vi "DblMonoPMDCurrentScan.vi"() -> ()   [LabVIEW 2009]
uses:
  <vilib>/DAQmx/create/channels.llb/DAQmx Create Channel (AI-Voltage-Basic).vi
  <vilib>/DAQmx/create/channels.llb/DAQmx Create Channel (AO-Voltage-Basic).vi
  <vilib>/DAQmx/write.llb/DAQmx Write (Analog DBL 1Chan 1Samp).vi
  <vilib>/DAQmx/read.llb/DAQmx Read (Analog 1D DBL 1Chan NSamp).vi
  <vilib>/DAQmx/configure/timing.llb/DAQmx Timing (Sample Clock).vi
  <vilib>/Utility/file.llb/Write To Spreadsheet File (DBL).vi
  <vilib>/Analysis/NI_AALBase.lvlib
panel:
  in  "PM Channel":refnum<visa-resource-name>="USB0::0x1313::0x8072::P2000362::INSTR"
  in  "Voltage B":dbl min=-10.0 max=10.0 step=0.1 format="%0.2f"
  in  "Voltage A":dbl min=-10.0 max=10.0 step=0.1 format="%0.2f"
  in  "Output B":tag="Dev1/ao3"
  in  "Output A":tag="Dev1/ao2"
  in  "Input Channel":tag="Dev1/ai6"
  in  "Current":bool
  in  "Power":bool=TRUE
  out "ScanGraph":cluster{dbl[], dbl[]}(graph)
  in  "Sensitivity":dbl=1e-09 caption="(A/V)" format="%#_6p"
  out "Readout":dbl=-5.1512643e-06 format="%^#_9e"
  in  "Scan Save Path":path
  in  "On":bool=TRUE
  out "Waveform Chart":dbl(graph)=-5.1512643e-06
  in  "Save":bool=TRUE
  in  "Exit":bool
  in  "STOP":bool
  in  "Step Time (sec)":dbl=1.0 min=0.001 max=300.0 step=0.001 format="%.3f"
  in  "Step Size (nm)":dbl=1.0 min=0.1 max=100.0 step=0.1 format="%.1f"
  in  "End":dbl=800.0 min=0.0 max=2000.0 step=0.1 format="%.1f"
  in  "Start":dbl=400.0 min=0.0 max=2000.0 step=0.1 format="%.1f"
  in  "Scan":bool
  in  "Up":bool=TRUE caption="Down"
  in  "Increment (nm)":dbl=10.0 min=0.1 max=2000.0 step=0.1 format="%.1f"
  in  "PMD Settings":T1={"Beam Diameter (mm)"=4.0, "BWIn"=0, "Averaging Rate"=300, "Auto Range"=TRUE} {"Averaging Rate" min=33 max=5000 step=1; "BWIn" items=["HIGH", "LOW"]; "Beam Diameter (mm)" min=1.0 max=9.0 step=0.5}
  in  "Step":bool
  out "Busy":bool
  in  "Send Command":bool
  in  "Command":u16(ring)=1 items=["nm", "goto", "nm/min", "VIS grating", "IR grating"]
  in  "Wavelength (nm)":dbl=500.0 min=0.0 max=2000.0 step=0.1 format="%.1f"
  in  "Scan Speed (nm/min)":dbl=100.0 min=1.0 max=500.0 step=0.1 format="%.1f"
  out "Done?":string="   ..."
  in  "Send Question":bool
  in  "Ask?":u16(ring) items=["?nm", "?nm/min", "?grating", "?turret", "?gratings"]
  in  "Zero?":bool
  out "PM Error log":string
  out "AUTO?":bool
  out "Zero Value":dbl format="%#.3p"
  out "Rng":string
  in  "Range":i16=1 min=1 max=6 step=1
  in  "Mono Port":refnum<visa-resource-name>="COM11"
  out "IDN String":string="Thorlabs,PM100USB,P2000362,1.3.0\n"
  out "Sensor SN":string="10061433"
  out "Sensor Name":string="S120C"
  out "Reply":string=" 0.000 nm  ok\r\n" caption="Mono Response"
  # "Range Settings"
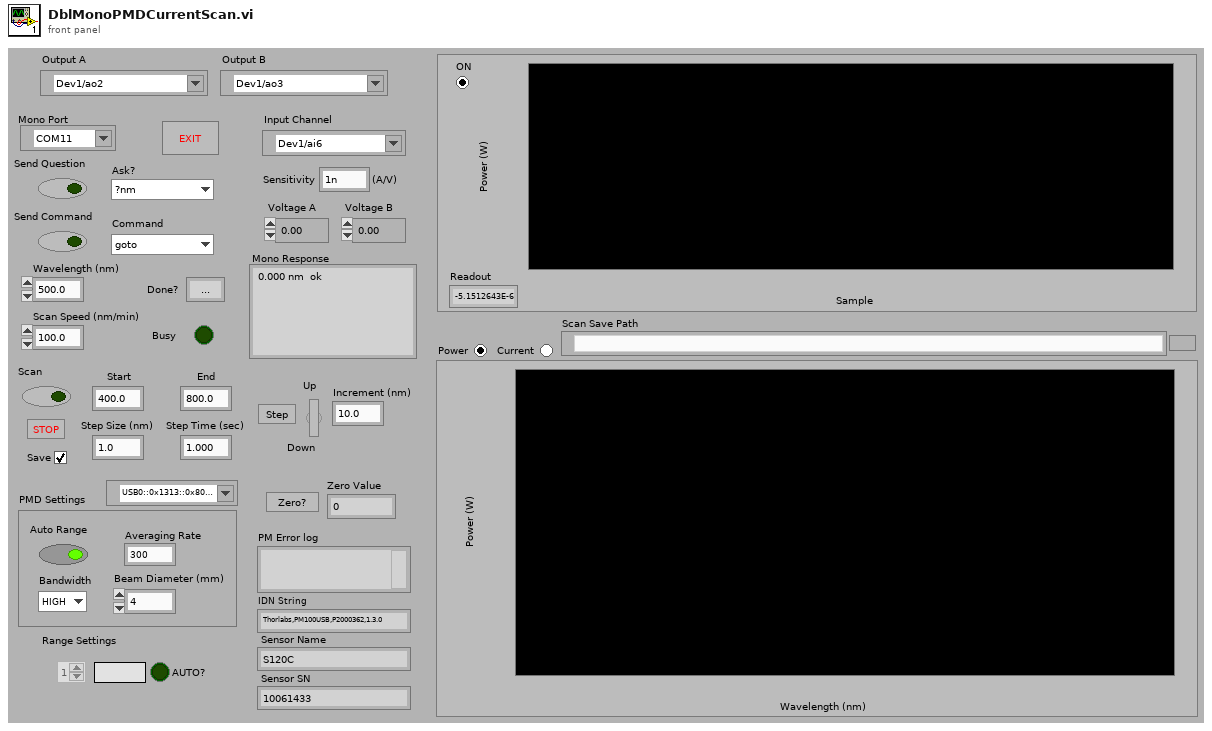
[diagram p1: front panel]
types:
  T1 = cluster{"Beam Diameter (mm)":dbl, "BWIn":u16, "Averaging Rate":i32, "Auto Range":bool}
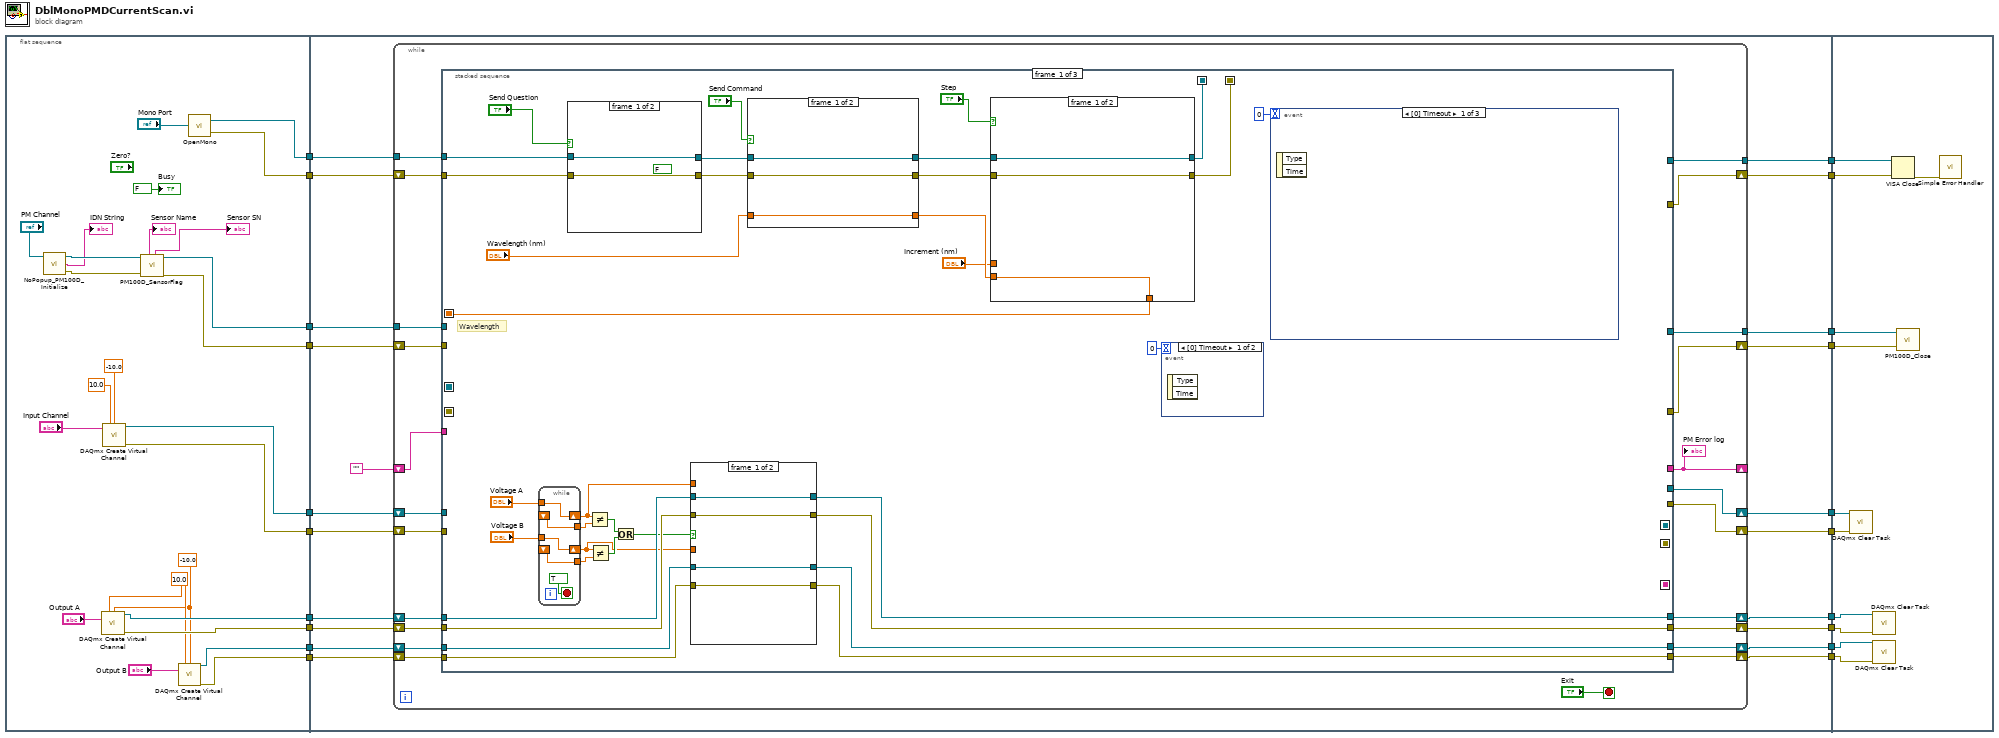
[diagram p0: block diagram]
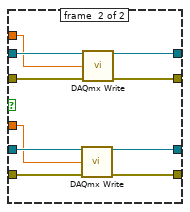
[diagram p2: hidden frame]
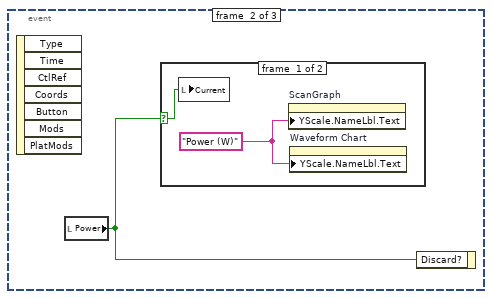
[diagram p3: hidden frame]
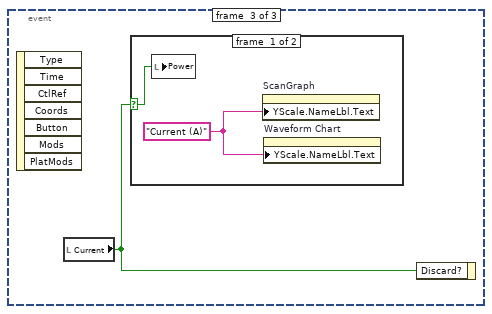
[diagram p5: hidden frame]
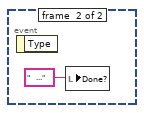
[diagram p7: hidden frame]
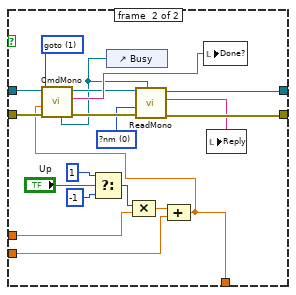
[diagram p8: hidden frame]
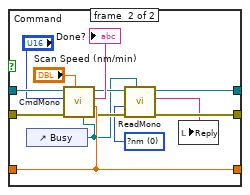
[diagram p9: hidden frame]
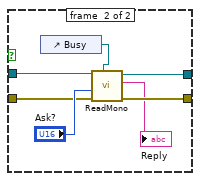
[diagram p10: hidden frame]
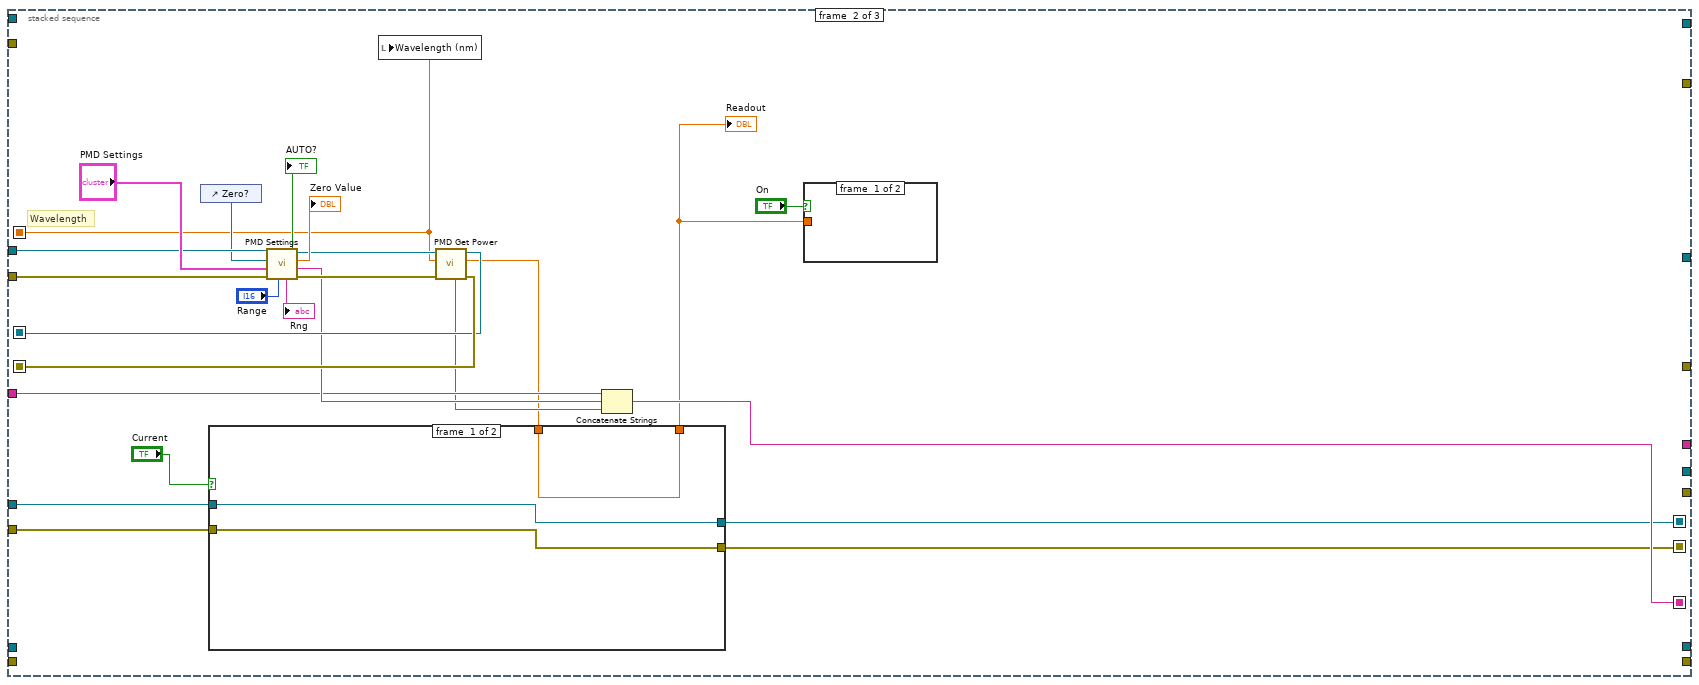
[diagram p11: hidden frame]
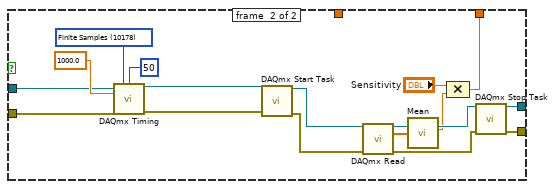
[diagram p12: hidden frame]
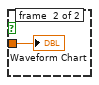
[diagram p13: hidden frame]
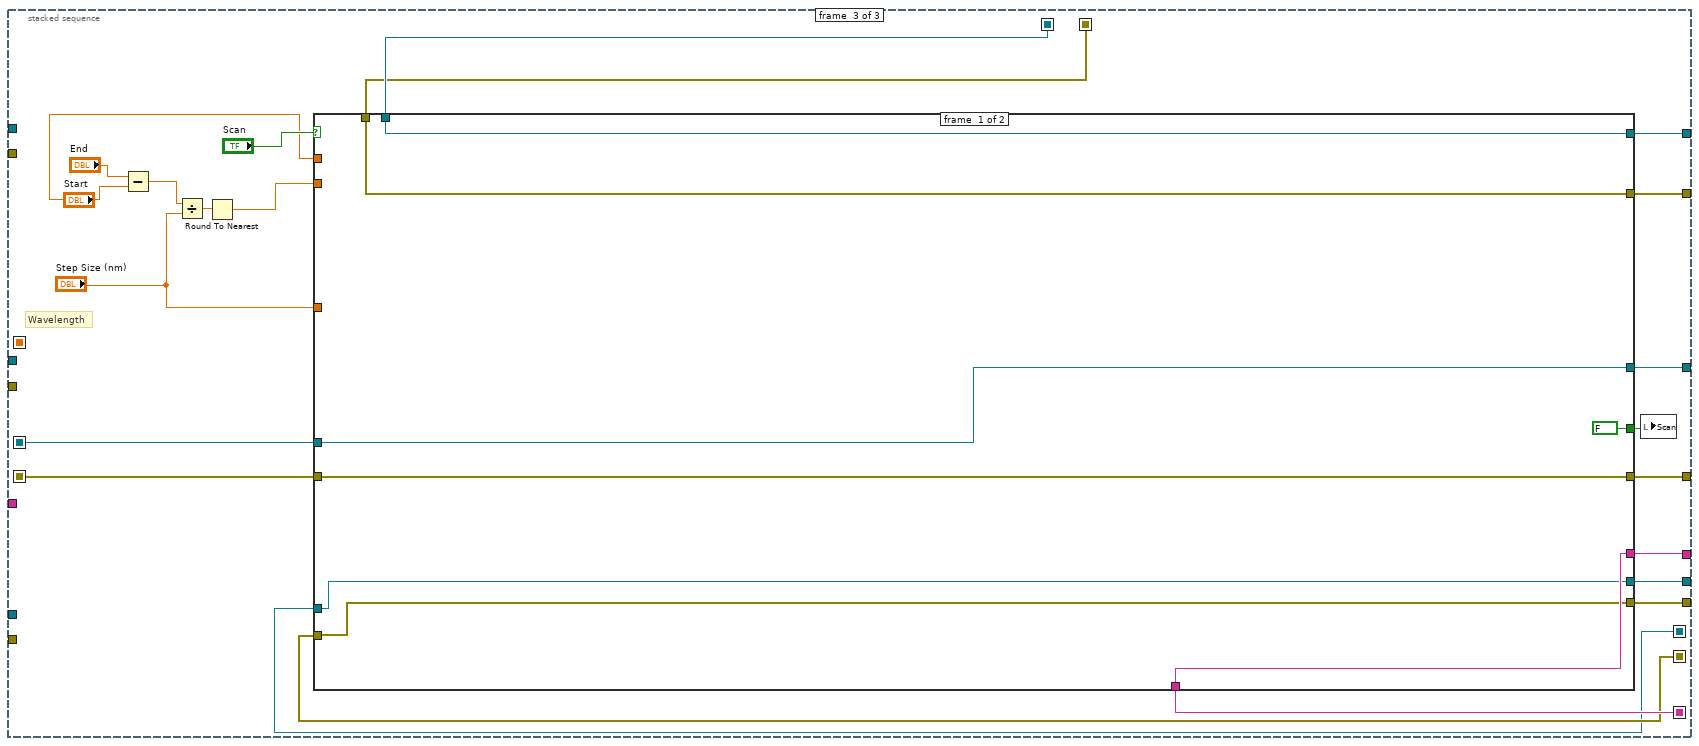
[diagram p14: hidden frame]
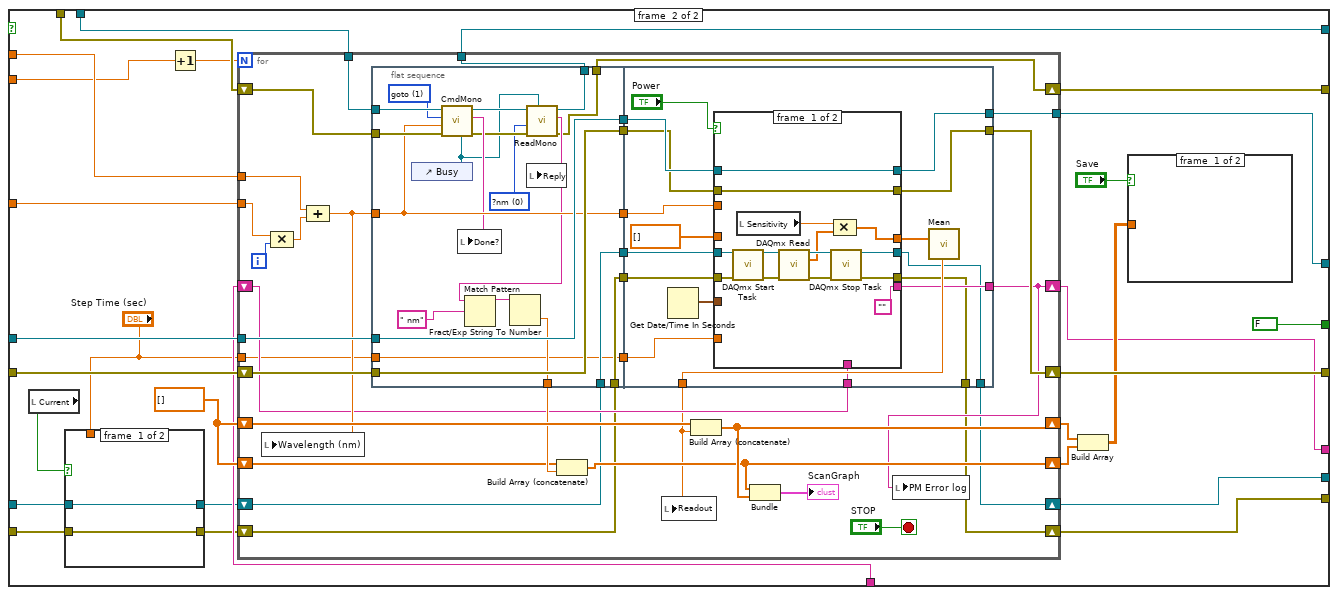
[diagram p15: hidden frame]
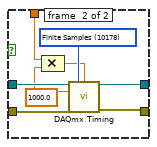
[diagram p16: hidden frame]
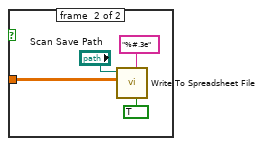
[diagram p17: hidden frame]
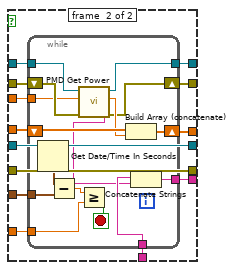
[diagram p18: hidden frame]
diagram:
  n1 = flat-sequence {
    tunnel: [w43] -> w20
    tunnel: [w42] -> w19
    tunnel: [w41] -> w18
    tunnel: [w40] -> w17
    tunnel: [w27] -> w12
    tunnel: [w28] -> w9
    tunnel: [w33] -> w8
    tunnel: [w34] -> w7
    tunnel: [w32] -> w6
    tunnel: [w31] -> w5
    tunnel: w20 -> [w65]
    tunnel: w19 -> [w66]
    tunnel: w18 -> [w64]
    tunnel: w17 -> [w63]
    tunnel: [w62] -> w16
    tunnel: [w61] -> w15
    tunnel: [w60] -> w14
    tunnel: [w59] -> w13
    tunnel: w12 -> [w56]
    tunnel: [w47] -> w11
    tunnel: [w46] -> w10
    tunnel: w9 -> [w57]
    tunnel: w8 -> [w55]
    tunnel: w7 -> [w54]
    tunnel: w6 -> [w53]
    tunnel: w5 -> [w52]
    tunnel: [w48] -> w4
    tunnel: [w49] -> w3
    tunnel: [w50] -> w2
    tunnel: [w51] -> w1
    tunnel: w16 -> [w438]
    tunnel: w15 -> [w437]
    tunnel: w14 -> [w436]
    tunnel: w13 -> [w435]
    tunnel: w11 -> [w433]
    tunnel: w10 -> [w434]
    tunnel: w4 -> [w432]
    tunnel: w3 -> [w431]
    tunnel: w2 -> [w430]
    tunnel: w1 -> [w429]
    frame #0 {
      w29 = -10.0 ("minimum value")
      w30 = 10.0 ("maximum value")
      n2 = call "NoPopup_PM100D_Initialize.vi"("PM Channel"="PM Channel") -> ("error out"=w23:errorcluster, "Instrument"=→"IDN String":string, "VISA out"=w24:refnum<visa-resource-name>)  [unwired: 1 in, 1 out]
      n3 = call-poly <vilib>:"DAQmx Create Virtual Channel.vi"("maximum value"=w30, "minimum value"=w29, "physical channels"="Output A") -> ("task out"=w34:refnum<k21>, "error out"=w33:errorcluster)  [unwired: 11 in]
      n4 = call-poly <vilib>:"DAQmx Create Virtual Channel.vi"("maximum value"=10.0, "minimum value"=-10.0, "physical channels"="Input Channel") -> ("task out"=w28:refnum<k21>, "error out"=w27:errorcluster)  [unwired: 11 in]
      n5 = call "PM100D_SensorFlag.vi"("error in (no error)"=w23, "VISA in"=w24) -> ("error out"=w43:errorcluster, "VISA out"=w42:refnum<visa-resource-name>, "sn"=→"Sensor SN":string, "name"=→"Sensor Name":string)  [unwired: 2 in, 4 out]
      n6 = call-poly <vilib>:"DAQmx Create Virtual Channel.vi"("maximum value"=w30, "minimum value"=w29, "physical channels"="Output B") -> ("task out"=w31:refnum<k21>, "error out"=w32:errorcluster)  [unwired: 11 in]
      n7 = call "OpenMono.vi"("Mono Port"="Mono Port") -> ("VISA resource name out"=w41:refnum<visa-resource-name>, "error out"=w40:errorcluster)
      "Busy" <- FALSE ("Busy")
    }
    frame #1 {
      n8 = while {
        tunnel: w66 -> [w87]
        tunnel: w64 -> [w89]
        tunnel: [w84] -> w61
        tunnel: [w82] -> w59
        shift-right: [w81] -> w60
        shift-left: w65 -> [w86]
        shift-right: [w83] -> w62
        shift-left: w63 -> [w88]
        shift-right: [w79] -> _
        shift-left: "" -> [w80]
        shift-right: [w68] -> w46
        shift-left: w56 -> [w77]
        shift-right: [w67] -> w47
        shift-left: w57 -> [w78]
        shift-right: [w69] -> w51
        shift-left: w54 -> [w76]
        shift-right: [w70] -> w50
        shift-left: w55 -> [w75]
        shift-right: [w71] -> w49
        shift-left: w52 -> [w73]
        shift-right: [w72] -> w48
        shift-left: w53 -> [w74]
        stop <- "Exit" stop-if-true
        n9 = stacked-sequence {
          seq-local: [w108 _ _] -> [_ w204 _]
          seq-local: [w113 _ _] -> [_ _ w257]
          seq-local: [w112 _ _] -> [_ _ w256]
          seq-local: [_ w211 _] -> [_ _ w255]
          seq-local: [_ w212 _] -> [_ _ w254]
          seq-local: [_ w205 _] -> [_ _ w248]
          seq-local: [_ w199 _] -> [_ _ w244]
          seq-local: [_ w200 _] -> [_ _ w243]
          tunnel: w89 -> [w119 _ _]
          tunnel: w88 -> [w118 _ _]
          tunnel: w87 -> [_ w214 _]
          tunnel: w86 -> [_ w213 _]
          tunnel: [_ _ w253] -> w84
          tunnel: [_ _ w252] -> w83
          tunnel: [_ _ w251] -> w82
          tunnel: [_ _ w250] -> w81
          tunnel: w80 -> [_ w207 _]
          tunnel: [_ _ w247] -> w79
          tunnel: w78 -> [_ w198 _]
          tunnel: w77 -> [_ w197 _]
          tunnel: [_ _ w246] -> w67
          tunnel: [_ _ w245] -> w68
          tunnel: w76 -> [w103 _ _]
          tunnel: w75 -> [w104 _ _]
          tunnel: w74 -> [w106 _ _]
          tunnel: w73 -> [w105 _ _]
          tunnel: [w102 _ _] -> w72
          tunnel: [w101 _ _] -> w71
          tunnel: [w100 _ _] -> w70
          tunnel: [w99 _ _] -> w69
          frame #0 {
            # "Wavelength"
            n10 = while {
              shift-right: [w141] -> w90
              shift-left: _ -> [w140]
              tunnel: "Voltage B" -> [w141]
              tunnel: [w140] -> w95
              tunnel: "Voltage A" -> [w139]
              shift-right: [w139] -> w91
              shift-left: _ -> [w138]
              tunnel: [w138] -> w96
              stop <- TRUE stop-if-true
            }
            n11 = case shown="True" "Send Question" {
              tunnel: w119 -> [w189 w195]
              tunnel: w118 -> [w188 w194]
              tunnel: [w189 w193] -> w121
              tunnel: [w188 w192] -> w120
              frame #0 {
                (unwired) FALSE ("Read Error")
              }
              frame #1 {
                n12 = control-ref of="Busy"() -> (w190:refnum<vi>)
                n13 = call "ReadMono.vi"("Busy"=w190, "error in (no error)"=w194, "Cmd"="Ask?", "Mono Port"=w195) -> ("error out"=w192:errorcluster, "Response"=→"Reply":string, "Mono Port Out"=w193:refnum<visa-resource-name>)  [unwired: 2 in, 1 out]
              }
            }
            n14 = Not Equal?(x=w91, y=w96) -> (x != y?=w94:bool)
            n15 = Not Equal?(x=w90, y=w95) -> (x != y?=w93:bool)
            n16 = Or(x=w94, y=w93) -> (x .or. y?=w92:bool)
            n17 = case shown="True" w92 {
              tunnel: w106 -> [w124 w137]
              tunnel: w105 -> [w125 w136]
              tunnel: w104 -> [w126 w135]
              tunnel: w103 -> [w127 w134]
              tunnel: [w124 w133] -> w102
              tunnel: [w125 w132] -> w101
              tunnel: [w126 w131] -> w100
              tunnel: [w127 w130] -> w99
              tunnel: w91 -> [_ w128]
              tunnel: w90 -> [_ w129]
              frame #0 {
              }
              frame #1 {
                n18 = call-poly <vilib>:"DAQmx Write.vi"("task/channels in"=w136, "data"=w129, "error in"=w137) -> ("task out"=w132:refnum<k21>, "error out"=w133:errorcluster)  [unwired: 10 in, 1 out]
                n19 = call-poly <vilib>:"DAQmx Write.vi"("task/channels in"=w134, "data"=w128, "error in"=w135) -> ("task out"=w130:refnum<k21>, "error out"=w131:errorcluster)  [unwired: 10 in, 1 out]
              }
            }
            n20 = case shown="True" "Send Command" {
              tunnel: w121 -> [w174 w187]
              tunnel: w120 -> [w173 w186]
              tunnel: [w174 w179] -> w116
              tunnel: [w173 w178] -> w115
              tunnel: "Wavelength (nm)" -> [w172 w182]
              tunnel: [w172 w182] -> w114
              frame #0 {
              }
              frame #1 {
                w177 = u16 0 items=["?nm", "?nm/min", "?grating", "?turret", "?gratings"] ("Cmd")
                n21 = control-ref of="Busy"() -> (w175:refnum<vi>)
                n22 = call "CmdMono.vi"("Busy"=w175, "Scan Speed (nm/min)"="Scan Speed (nm/min)", "error in (no error)"=w186, "Wavelength (nm)"=w182, "Cmd"="Command", "Mono Port"=w187) -> ("error out"=w180:errorcluster, "Response"=→"Done?":string, "Mono Port Out"=w181:refnum<visa-resource-name>)  [unwired: 2 in, 1 out]
                n23 = call "ReadMono.vi"("Busy"=w175, "error in (no error)"=w180, "Cmd"=w177, "Mono Port"=w181) -> ("error out"=w178:errorcluster, "Response"=w176:string, "Mono Port Out"=w179:refnum<visa-resource-name>)  [unwired: 2 in, 1 out]
                n24 = local write "Reply"(w176) -> ()
              }
            }
            n25 = case shown="False" "Step" {
              tunnel: w116 -> [w152 w171]
              tunnel: w115 -> [w151 w170]
              tunnel: w114 -> [w150 w164]
              tunnel: [w152 w157] -> w113
              tunnel: [w151 w158] -> w112
              tunnel: "Increment (nm)" -> [_ w163]
              tunnel: [w150 w153] -> w108
              frame #0 {
              }
              frame #1 {
                w155 = u16 0 items=["?nm", "?nm/min", "?grating", "?turret", "?gratings"] ("Cmd")
                w162 = u16 1 items=["nm", "goto", "nm/min", "VIS grating", "IR grating"] ("Cmd")
                n26 = Select(t=1, s="Up", f=-1) -> (s? t:f=w169:i32)
                n27 = control-ref of="Busy"() -> (w154:refnum<vi>)
                n28 = Compound Arithmetic op=MULTIPLY(w169, w163) -> (w165:dbl)
                n29 = Compound Arithmetic op=ADD(w165, w164) -> (w153:dbl)
                n30 = call "CmdMono.vi"("Busy"=w154, "error in (no error)"=w170, "Wavelength (nm)"=w153, "Cmd"=w162, "Mono Port"=w171) -> ("error out"=w159:errorcluster, "Response"=w161:string, "Mono Port Out"=w160:refnum<visa-resource-name>)  [unwired: 3 in, 1 out]
                n31 = call "ReadMono.vi"("Busy"=w154, "error in (no error)"=w159, "Cmd"=w155, "Mono Port"=w160) -> ("error out"=w158:errorcluster, "Response"=w156:string, "Mono Port Out"=w157:refnum<visa-resource-name>)  [unwired: 2 in, 1 out]
                n32 = local write "Done?"(w161) -> ()
                n33 = local write "Reply"(w156) -> ()
              }
            }
            n34 = event shown="[0] Timeout" {
              selector: _ -> [_ _]
              dyn-events: _ -> [_ _]
              timeout: 0 -> [_ _]
              event #0 {
                n35 = event-data() -> ()  [unwired: 1 in, 2 out]
              }
              event #1 {
                n36 = event-data() -> ()  [unwired: 1 in, 1 out]
                n37 = local write "Done?"("   ..." ("Done?")) -> ()
              }
            }
            n38 = event shown="[0] Timeout" {
              selector: _ -> [_ _ _]
              dyn-events: _ -> [_ _ _]
              timeout: 0 -> [_ _ _]
              event #0 {
                n39 = event-data() -> ()  [unwired: 1 in, 2 out]
              }
              event #1 {
                n40 = event-data() -> ()  [unwired: 1 in, 7 out]
                n41 = local read "Power"() -> (w143:bool)
                n42 = case shown="False" w143 {
                  selector: w143 -> [w145 _]
                  frame #0 {
                    w144 = "Power (W)" ("Y Scale.Name Label.Text")
                    n43 = local write "Current"(w145) -> ()
                    n44 = property on="ScanGraph" class="XYGraph (strict)"("YScale.NameLbl.Text"=w144) -> ()  [unwired: 2 in, 2 out]
                    n45 = property on="Waveform Chart" class="WFChart (strict)"("YScale.NameLbl.Text"=w144) -> ()  [unwired: 2 in, 2 out]
                  }
                  frame #1 {
                  }
                }
                n46 = event-data("Discard?"=w143) -> ()  [unwired: 1 in, 1 out]
              }
              event #2 {
                n47 = event-data() -> ()  [unwired: 1 in, 7 out]
                n48 = local read "Current"() -> (w146:bool)
                n49 = case shown="False" w146 {
                  selector: w146 -> [w147 _]
                  frame #0 {
                    w148 = "Current (A)" ("Y Scale.Name Label.Text")
                    n50 = local write "Power"(w147) -> ()
                    n51 = property on="ScanGraph" class="XYGraph (strict)"("YScale.NameLbl.Text"=w148) -> ()  [unwired: 2 in, 2 out]
                    n52 = property on="Waveform Chart" class="WFChart (strict)"("YScale.NameLbl.Text"=w148) -> ()  [unwired: 2 in, 2 out]
                  }
                  frame #1 {
                  }
                }
                n53 = event-data("Discard?"=w146) -> ()  [unwired: 1 in, 1 out]
              }
            }
          }
          frame #1 {
            # "Wavelength"
            n54 = control-ref of="Zero?"() -> (w209:refnum<vi>)
            n55 = call "PMD Settings.vi"("Visa In"=w214, "Zero?"=w209, "PMD Settings In"="PMD Settings", "Error In"=w213, "Range"="Range") -> ("AUTO?"=→"AUTO?":bool, "Rng"=→"Rng":string, "Visa Out"=w217:refnum<visa-resource-name>, "ZeroValue"=→"Zero Value":dbl, "PM Error log"=w208:string, "error out"=w216:errorcluster)
            n56 = local write "Wavelength (nm)"(w204) -> ()
            n57 = call "PMD Get Power.vi"("VISA In"=w217, "Wavelength (nm)"=w204, "error in"=w216) -> ("PMD Error"=w206:string, "VISA out"=w211:refnum<visa-resource-name>, "Readout value"=w203:dbl, "error out"=w212:errorcluster)  [unwired: 1 in, 2 out]
            n58 = case shown="False" "Current" {
              tunnel: w203 -> [w224 _]
              tunnel: w198 -> [w223 w227]
              tunnel: w197 -> [w222 w228]
              tunnel: [w224 w240] -> w201
              tunnel: [w222 w236] -> w199
              tunnel: [w223 w237] -> w200
              frame #0 {
              }
              frame #1 {
                w230 = 10178 items=["Finite Samples"=10178, "Continuous Samples"=10123, "Hardware Timed Single Point"=12522] ("sample mode")
                n59 = call-poly <vilib>:"DAQmx Timing.vi"("task/channels in"=w227, "sample mode"=w230, "samples per channel"=50, "rate"=1000.0, "error in"=w228) -> ("task out"=w226:refnum<k21>, "error out"=w225:errorcluster)  [unwired: 9 in]
                n60 = call <vilib>:"DAQmx Start Task.vi"("task/channels in"=w226, "error in"=w225) -> ("task out"=w238:refnum<k21>, "error out"=w239:errorcluster)  [unwired: 12 in]
                n61 = call-poly <vilib>:"DAQmx Read.vi"("task/channels in"=w238, "error in"=w239) -> ("task out"=w234:refnum<k21>, "data"=w233:dbl[], "error out"=w235:errorcluster)  [unwired: 11 in]
                n62 = call <vilib>:"Mean.vi"("X"=w233) -> ("mean"=w232:dbl)  [unwired: 1 out]
                n63 = Compound Arithmetic op=MULTIPLY("Sensitivity", w232) -> (w240:dbl)
                n64 = call <vilib>:"DAQmx Stop Task.vi"("task/channels in"=w234, "error in"=w235) -> ("task out"=w237:refnum<k21>, "error out"=w236:errorcluster)  [unwired: 12 in]
              }
            }
            "Readout" <- w201
            n65 = Concatenate Strings(w207, w208, w206) -> (w205:string)
            n66 = case shown="True" "On" {
              tunnel: w201 -> [_ w242]
              frame #0 {
              }
              frame #1 {
                "Waveform Chart" <- w242
              }
            }
          }
          frame #2 {
            # "Wavelength"
            n67 = Subtract(x="End", y="Start") -> (x-y=w262:dbl)
            n68 = Divide(x=w262, y="Step Size (nm)") -> (x/y=w261:dbl)
            n69 = Round To Nearest(number=w261) -> (nearest integer value=w260:dbl)
            n70 = case shown="False" "Scan" {
              tunnel: w260 -> [_ w295]
              tunnel: w256 -> [w270 w297]
              tunnel: w257 -> [w269 w298]
              tunnel: "Start" -> [_ w300]
              tunnel: "Step Size (nm)" -> [_ w299]
              tunnel: w255 -> [w272 w293]
              tunnel: w254 -> [w271 w292]
              tunnel: [w272 w281] -> w251
              tunnel: [w271 w291] -> w250
              tunnel: [w270 w290] -> w252
              tunnel: [w269 w289] -> w253
              tunnel: [FALSE ("Scan") FALSE ("Scan")] -> w249
              tunnel: w248 -> [w267 w283]
              tunnel: [w267 w282] -> w247
              tunnel: [w266 w280] -> w246
              tunnel: [w265 w279] -> w245
              tunnel: w244 -> [w265 w277]
              tunnel: w243 -> [w266 w276]
              frame #0 {
              }
              frame #1 {
                w296 = dbl[] []
                n71 = local read "Current"() -> (w278:bool)
                n72 = case shown="True" w278 {
                  tunnel: w277 -> [w301 w309]
                  tunnel: w276 -> [w302 w308]
                  tunnel: [w302 w307] -> w275
                  tunnel: [w301 w306] -> w274
                  tunnel: "Step Time (sec)" -> [_ w305]
                  frame #0 {
                  }
                  frame #1 {
                    w310 = 10178 items=["Finite Samples"=10178, "Continuous Samples"=10123, "Hardware Timed Single Point"=12522] ("sample mode")
                    w304 = 1000.0 ("rate")
                    n73 = Compound Arithmetic op=MULTIPLY(w305, w304) -> (w303:dbl)
                    n74 = call-poly <vilib>:"DAQmx Timing.vi"("task/channels in"=w308, "sample mode"=w310, "samples per channel"=w303, "rate"=w304, "error in"=w309) -> ("task out"=w307:refnum<k21>, "error out"=w306:errorcluster)  [unwired: 9 in]
                  }
                }
                n75 = Increment(x=w295) -> (x+1=w294:dbl)
                n76 = for {
                  N: w294 -> [_]
                  tunnel: w298 -> [w346]
                  tunnel: w300 -> [w342]
                  tunnel: w299 -> [w344]
                  shift-right: [w330] -> w288
                  shift-left: w296 -> [w348]
                  shift-right: [w341] -> w290
                  shift-left: w297 -> [w347]
                  shift-right: [w326] -> w287
                  shift-left: w296 -> [w327]
                  tunnel: w293 -> [w339]
                  shift-right: [w334] -> w291
                  shift-left: w292 -> [w338]
                  tunnel: [w333] -> w281
                  tunnel: [w332] -> w289
                  shift-right: [w324] -> w282
                  shift-left: w283 -> [w325]
                  shift-right: [w321] -> w279
                  shift-left: w274 -> [w316]
                  shift-right: [w320] -> w280
                  shift-left: w275 -> [w317]
                  tunnel: "Step Time (sec)" -> [w318]
                  i -> [w345]
                  stop <- "STOP" stop-if-true
                  n77 = Compound Arithmetic op=MULTIPLY(w344, w345) -> (w343:dbl)
                  n78 = Compound Arithmetic op=ADD(w342, w343) -> (w329:dbl)
                  n79 = local write "Wavelength (nm)"(w329) -> ()
                  n80 = flat-sequence {
                    tunnel: w347 -> [w368]
                    tunnel: w346 -> [w367]
                    tunnel: w329 -> [w363]
                    tunnel: [w352] -> w341
                    tunnel: w339 -> [w365]
                    tunnel: w338 -> [w364]
                    tunnel: [w365] -> w337
                    tunnel: [w364] -> w336
                    tunnel: [w363] -> w335
                    tunnel: [w357] -> w332
                    tunnel: [w353] -> w328
                    tunnel: w316 -> [w350]
                    tunnel: [w351] -> w323
                    tunnel: w317 -> [w351]
                    tunnel: [w350] -> w322
                    tunnel: [w349] -> w319
                    tunnel: w318 -> [w349]
                    tunnel: [w382] -> w315
                    tunnel: w337 -> [w381]
                    tunnel: w336 -> [w380]
                    tunnel: w335 -> [w379]
                    tunnel: [w375] -> w334
                    tunnel: [w378] -> w333
                    tunnel: w325 -> [w377]
                    tunnel: [w376] -> w324
                    tunnel: w323 -> [w373]
                    tunnel: w322 -> [w372]
                    tunnel: [w370] -> w320
                    tunnel: [w371] -> w321
                    tunnel: w319 -> [w374]
                    frame #0 {
                      w359 = u16 0 items=["?nm", "?nm/min", "?grating", "?turret", "?gratings"] ("Cmd")
                      w366 = u16 1 items=["nm", "goto", "nm/min", "VIS grating", "IR grating"] ("Cmd")
                      n81 = control-ref of="Busy"() -> (w358:refnum<vi>)
                      n82 = call "CmdMono.vi"("Busy"=w358, "error in (no error)"=w368, "Wavelength (nm)"=w363, "Cmd"=w366, "Mono Port"=w367) -> ("error out"=w360:errorcluster, "Response"=w362:string, "Mono Port Out"=w361:refnum<visa-resource-name>)  [unwired: 3 in, 1 out]
                      n83 = local write "Done?"(w362) -> ()
                      n84 = call "ReadMono.vi"("Busy"=w358, "error in (no error)"=w360, "Cmd"=w359, "Mono Port"=w361) -> ("error out"=w352:errorcluster, "Response"=w355:string, "Mono Port Out"=w357:refnum<visa-resource-name>)  [unwired: 2 in, 1 out]
                      n85 = Match Pattern(string=w355, regular expression=" nm") -> (before substring=w354:string)  [unwired: 1 in, 3 out]
                      n86 = Fract/Exp String To Number(string=w354) -> (number=w353:dbl)  [unwired: 3 in, 1 out]
                      n87 = local write "Reply"(w355) -> ()
                    }
                    frame #1 {
                      n88 = Get Date/Time In Seconds() -> (seconds since 1Jan1904=w384:timestamp)
                      n89 = case shown="True" "Power" {
                        tunnel: dbl[] [] -> [_ w412]
                        tunnel: w384 -> [_ w411]
                        tunnel: [w386 w410] -> w383
                        tunnel: w381 -> [w398 w409]
                        tunnel: w380 -> [w397 w408]
                        tunnel: w379 -> [_ w407]
                        tunnel: [w398 w406] -> w378
                        tunnel: w377 -> [_ w405]
                        tunnel: ["" w404] -> w376
                        tunnel: [w397 w403] -> w375
                        tunnel: w374 -> [_ w402]
                        tunnel: w373 -> [w396 w400]
                        tunnel: w372 -> [w395 w401]
                        tunnel: [w390 w401] -> w371
                        tunnel: [w389 w400] -> w370
                        frame #0 {
                          n90 = call <vilib>:"DAQmx Start Task.vi"("task/channels in"=w396, "error in"=w395) -> ("task out"=w394:refnum<k21>, "error out"=w393:errorcluster)  [unwired: 12 in]
                          n91 = local read "Sensitivity"() -> (w387:dbl)
                          n92 = call-poly <vilib>:"DAQmx Read.vi"("task/channels in"=w394, "error in"=w393) -> ("task out"=w392:refnum<k21>, "data"=w388:dbl[], "error out"=w391:errorcluster)  [unwired: 11 in]
                          n93 = call <vilib>:"DAQmx Stop Task.vi"("task/channels in"=w392, "error in"=w391) -> ("task out"=w389:refnum<k21>, "error out"=w390:errorcluster)  [unwired: 12 in]
                          n94 = Compound Arithmetic op=MULTIPLY(w387, w388) -> (w386:dbl[])
                        }
                        frame #1 {
                          n95 = while {
                            shift-right: [w427] -> w410
                            shift-left: w412 -> [w428]
                            tunnel: w411 -> [w425]
                            tunnel: w409 -> [w420]
                            tunnel: w407 -> [w416]
                            tunnel: [w418] -> w406
                            tunnel: w405 -> [w422]
                            tunnel: [w421] -> w404
                            shift-right: [w414] -> w403
                            shift-left: w408 -> [w419]
                            tunnel: w402 -> [w413]
                            stop <- w423 stop-if-true
                            n96 = Get Date/Time In Seconds() -> (seconds since 1Jan1904=w426:timestamp)
                            n97 = Subtract(x=w426, y=w425) -> (x-y=w424:dbl)
                            n98 = call "PMD Get Power.vi"("VISA In"=w420, "Wavelength (nm)"=w416, "error in"=w419) -> ("PMD Error"=w415:string, "VISA out"=w418:refnum<visa-resource-name>, "Readout value"=w417:dbl, "error out"=w414:errorcluster)  [unwired: 1 in, 2 out]
                            n99 = Greater Or Equal?(x=w424, y=w413) -> (x >= y?=w423:bool)
                            n100 = Build Array (concatenate)(w428, w417) -> (w427:dbl[])
                            n101 = Concatenate Strings(w422, w415) -> (w421:string)
                          }
                        }
                      }
                      n102 = call <vilib>:"Mean.vi"("X"=w383) -> ("mean"=w382:dbl)  [unwired: 1 out]
                    }
                  }
                  n103 = Build Array (concatenate)(w327, w328) -> (w326:dbl[])
                  n104 = local write "Readout"(w315) -> ()
                  n105 = Build Array (concatenate)(w348, w315) -> (w330:dbl[])
                  n106 = Bundle(w326, w330) -> (→"ScanGraph":cluster{dbl[], dbl[]})  [unwired: 1 in]
                  n107 = local write "PM Error log"(w324) -> ()
                }
                n108 = Build Array(w288, w287) -> (w286:dbl[][])
                n109 = case shown="True" "Save" {
                  tunnel: w286 -> [_ w311]
                  frame #0 {
                  }
                  frame #1 {
                    n110 = call-poly <vilib>:"Write To Spreadsheet File.vi"("transpose? (no:F)"=TRUE, "format (%.3f)"="%#.3e", "2D data"=w311, "file path (dialog if empty)"="Scan Save Path") -> ()  [unwired: 4 in, 1 out]
                  }
                }
              }
            }
            n111 = local write "Scan"(w249) -> ()
          }
        }
        "PM Error log" <- w79
      }
    }
    frame #2 {
      n112 = call <vilib>:"DAQmx Clear Task.vi"("task in"=w433, "error in"=w434) -> ()  [unwired: 13 in, 1 out]
      n113 = call <vilib>:"DAQmx Clear Task.vi"("task in"=w429, "error in"=w430) -> ()  [unwired: 13 in, 1 out]
      n114 = call <vilib>:"DAQmx Clear Task.vi"("task in"=w431, "error in"=w432) -> ()  [unwired: 13 in, 1 out]
      n115 = VISA Close(VISA resource name=w437, error in (no error)=w438) -> (error out=w439:errorcluster)
      n116 = call "PM100D_Close.vi"("error in (no error)"=w436, "VISA resource name"=w435) -> ()  [unwired: 2 in]
      n117 = call <vilib>:"Simple Error Handler.vi"("error in (no error)"=w439) -> ()  [unwired: 1 in, 8 out]
    }
  }
